vi "Log Message.vi"(6 "Ack Requested":bool, 8 "error in":errorcluster, 9 "Module Action":string, 10 "Message Data In":variant, 11 "Module Data In":refnum<class "Rename.lvclass">) -> (0 "error out":errorcluster, 1 "Module Action":string, 2 "Message Data Out":variant, 3 "Module Data Out":refnum<class "Rename.lvclass">)   [LabVIEW 2015, in "Generic Module Library.lvlib" / "Template G_Module.lvlib"]
uses:
  Template G_Module.lvlib
  Module Class/Rename.lvclass
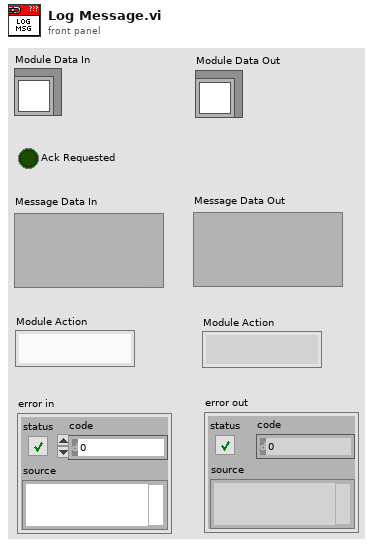
[diagram p1: front panel]
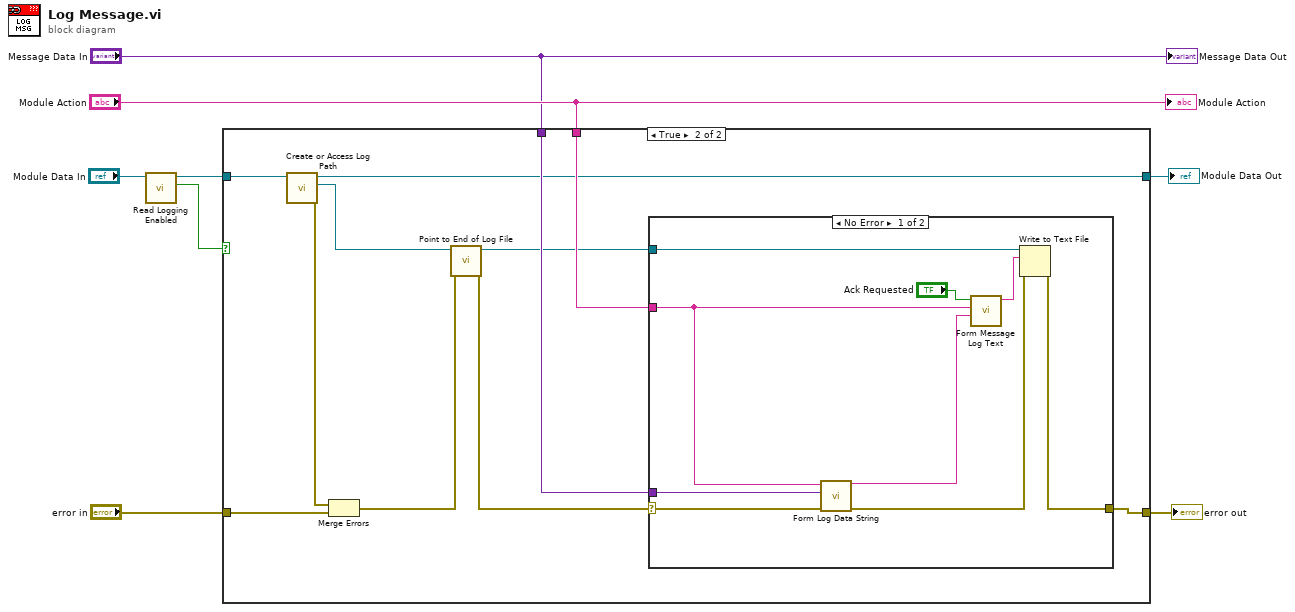
[diagram p0: block diagram]
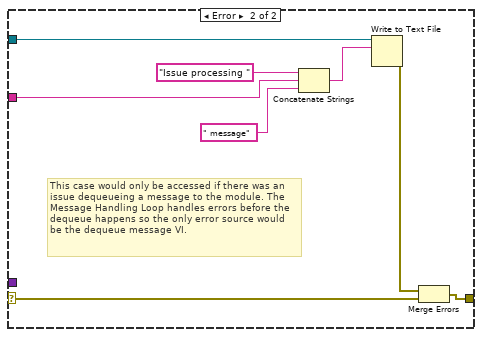
[diagram p3: hidden frame]
diagram:
  n1 = call-dynamic "Read Logging Enabled.vi"("Rename in"="Module Data In") -> ("Logging Enabled"=w2:bool, "Rename out"=w3:refnum<class "Rename.lvclass">)  [unwired: 8 in, 1 out]
  n2 = case shown="True" w2 {
    tunnel: [w10 w21] -> w8
    tunnel: "error in" -> [w10 w20]
    tunnel: "Module Action" -> [_ w18]
    tunnel: "Message Data In" -> [_ w17]
    tunnel: w3 -> [w9 w12]
    tunnel: [w9 w11] -> w1
    frame False {
    }
    frame True {
      n3 = call "Create or Access Log Path.vi"("Module Data In"=w12) -> ("error out"=w19:errorcluster, "Log Refnum Out"=w16:refnum<file>, "Module Data Out"=w11:refnum<class "Rename.lvclass">)  [unwired: 7 in, 1 out]
      n4 = Merge Errors(w19, w20) -> (w14:errorcluster)
      n5 = call "Point to End of Log File.vi"("error in (no error)"=w14, "Byte Stream File in"=w16) -> ("error out"=w13:errorcluster, "Byte Stream File out"=w15:refnum<file>)  [unwired: 8 in]
      n6 = case shown="No Error" w13 {
        selector: w13 -> [w26 w34]
        tunnel: w15 -> [w27 w38]
        tunnel: [w30 w36] -> w21
        tunnel: w18 -> [w29 w31]
        tunnel: w17 -> [w28 _]
        frame No Error {
          n7 = call "Form Log Data String.vi"("error in (no error)"=w26, "Message Data In"=w28, "Log Text"=w29) -> ("error out"=w23:errorcluster, "Log Data String"=w22:string)  [unwired: 7 in]
          n8 = call "Form Message Log Text.vi"("Data String Input"=w22, "Module Action"=w29, "Ack Requested"="Ack Requested") -> ("String to Write"=w25:string)  [unwired: 8 in]
          n9 = Write to Text File(file (use dialog)=w27, text=w25, error in=w23) -> (error out=w30:errorcluster)  [unwired: 1 in, 2 out]
        }
        frame Error {
          # "This case would only be accessed if there was an issue dequeueing a message to the module. The Message Handling Loop handles errors before the dequeue happens so the only error source would be the dequeue message VI."
          n10 = Concatenate Strings("Issue processing " ("string"), w31, " message" ("string")) -> (w37:string)
          n11 = Write to Text File(file (use dialog)=w38, text=w37) -> (error out=w35:errorcluster)  [unwired: 2 in, 2 out]
          n12 = Merge Errors(w35, w34) -> (w36:errorcluster)
        }
      }
    }
  }
  "error out" <- w8
  "Module Data Out" <- w1
  "Message Data Out" <- "Message Data In"
  "Module Action" <- "Module Action"
